vi "Write.vi"(8 "error in (no error)":errorcluster, 10 "Input":variant, 11 "DAQmx AI in":refnum<class "DAQmx AI.lvclass">) -> (0 "error out":errorcluster, 3 "DAQmx AI out":refnum<class "DAQmx AI.lvclass">)   [LabVIEW 2017, in "DAQmx AI.lvclass"]
uses:
  DAQmx AI.lvclass
  DAQmx/DAQmx.lvclass
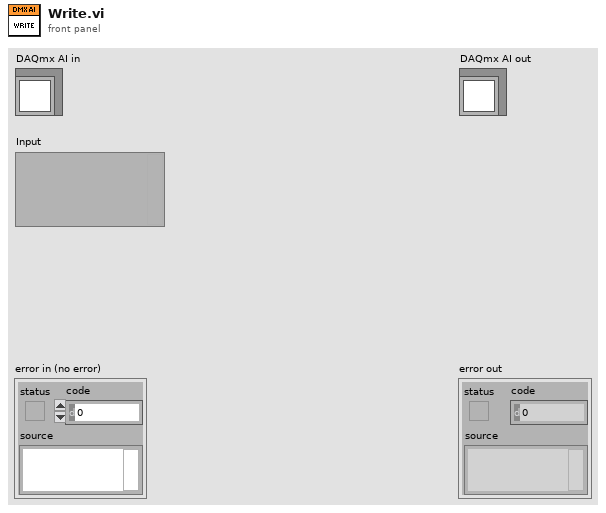
[diagram p1: front panel]
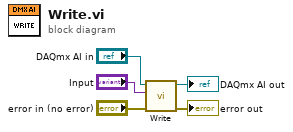
[diagram p0: block diagram]
diagram:
  n1 = call-parent "Write.vi"("error in (no error)"="error in (no error)", "Input"="Input", "DAQmx in"="DAQmx AI in") -> ("error out"=→"error out":errorcluster, "DAQmx out"=→"DAQmx AI out":refnum<class "DAQmx AI.lvclass">)  [unwired: 7 in]
